vi "Current Elevator State.vi"(8 "error in (no error)":errorcluster, 10 "Elevator State":T1 {"Current Elevation" scale=0.0..100.0; "Current Travel Rate" scale=-1.0..1.0}, 11 "GTH-Assessing in":refnum<class "GTH-Assessing.lvclass">) -> (0 "error out":errorcluster, 3 "GTH-Assessing out":refnum<class "GTH-Assessing.lvclass">)   [LabVIEW 2014, in "Elevator.lvlib" / "EL-Go To Height.lvlib" / "GTH-Assessing.lvclass"]
uses:
  GTH-Assessing.lvclass
  Elevator Class/Elevator State.ctl
  <vilib>/ActorFramework/Actor/Actor.lvclass/Actor.ctl
  <vilib>/ActorFramework/Message Enqueuer/Message Enqueuer.lvclass/Message Enqueuer.ctl
  <vilib>/ActorFramework/Message Enqueuer/Init from Existing Queue.vi
  <vilib>/ActorFramework/Message Enqueuer/Enqueue.vi
  <vilib>/ActorFramework/Message Priority Queue/Priority Enqueue.vi
  <vilib>/ActorFramework/Message Enqueuer/Message Enqueuer.lvclass
  EL-Go To Height Messages/Go To Holding Msg/Go To Holding Msg.lvclass
  EL-Go To Height Messages/Go To Down Msg/Go To Down Msg.lvclass
  EL-Go To Height Messages/Go To Up Msg/Go To Up Msg.lvclass
  EL-Go To Height Class/EL-Go To Height.lvclass
  <vilib>/ActorFramework/Actor/Actor.lvclass
  Elevator Class/Elevator.lvclass
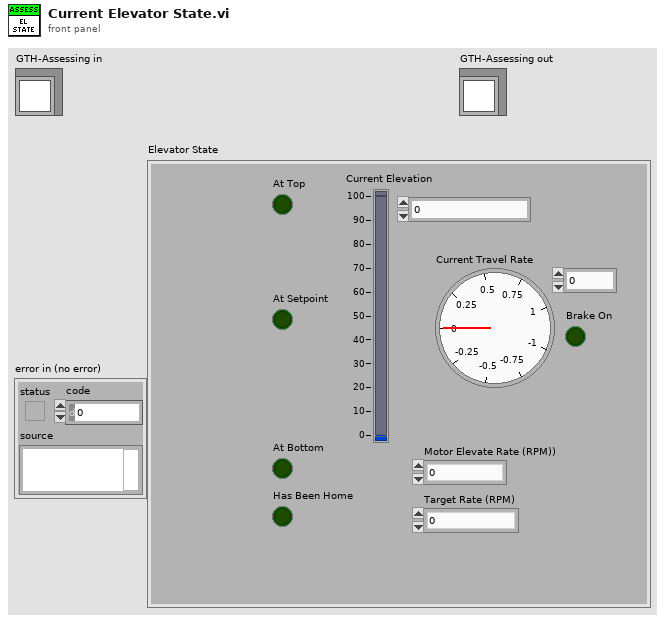
[diagram p1: front panel]
types:
  T1 = typedef "Elevator.lvlib/Elevator.lvclass/Elevator State.ctl" = cluster{"At Bottom":bool, "At Top":bool, "At Setpoint":bool, "Target Rate (RPM)":dbl, "Current Travel Rate":dbl, "Current Elevation":dbl, "Brake On":bool, "Motor Elevate Rate (RPM))":dbl, "Has Been Home":bool}
  T2 = typedef "Elevator.lvlib/EL-Go To Height.lvlib/EL-Go To Height.lvclass/Parameters.ctl" = cluster{"Target Height":dbl, "Elevator State Loop (ms)":u32, "Up Rate (Percentage)":dbl, "Down Rate (Percentage)":dbl}
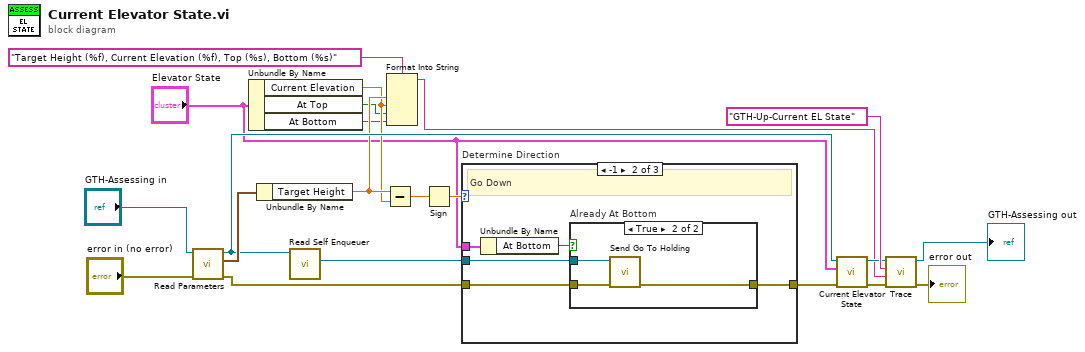
[diagram p0: block diagram]
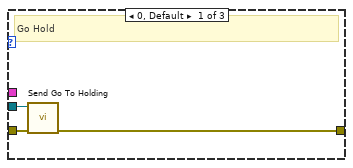
[diagram p2: hidden frame]
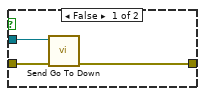
[diagram p3: hidden frame]
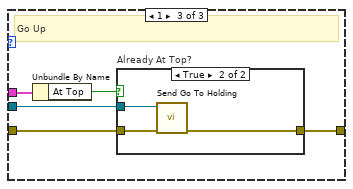
[diagram p4: hidden frame]
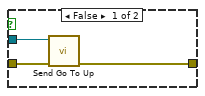
[diagram p5: hidden frame]
diagram:
  n1 = call-dynamic "Read Parameters.vi"("error in (no error)"="error in (no error)", "EL-Go To Height in"="GTH-Assessing in") -> ("error out"=w16:errorcluster, "Parameters"=w21:T2, "EL-Go To Height out"=w13:refnum<class "GTH-Assessing.lvclass">)  [unwired: 7 in]
  n2 = Unbundle By Name("Elevator State") -> ("Current Elevation"=w4:dbl, "At Top"=w2:bool, "At Bottom"=w1:bool)
  n3 = Unbundle By Name(w21) -> ("Target Height"=w5:dbl)
  n4 = call <vilib>:"Read Self Enqueuer.vi"("Actor"=w13) -> ("Self Enqueuer"=w18:refnum<class "Message Enqueuer.lvclass">)  [unwired: 10 in]
  n5 = Subtract(x=w5, y=w4) -> (x-y=w20:dbl)
  n6 = Format Into String(format string="Target Height (%f), Current Elevation (%f), Top (%s), Bottom (%s)", w5, w4, w2, w1) -> (resulting string=w6:string)  [unwired: 2 in, 1 out]
  n7 = Sign(1:w20) -> (0:w19:dbl)
  n8 = case "Determine Direction" shown="-1" w19 {
    tunnel: w18 -> [w24 w29 w38]
    tunnel: w16 -> [w23 w27 w37]
    tunnel: [w22 w28 w36] -> w15
    tunnel: "Elevator State" -> [_ w26 w40]
    frame 0, Default {
      # "Go Hold"
      n9 = call "Send Go To Holding.vi"("error in (no error)"=w23, "Message Enqueuer"=w24) -> ("error out"=w22:errorcluster)  [unwired: 8 in, 1 out]
    }
    frame -1 {
      # "Go Down"
      n10 = Unbundle By Name(w26) -> ("At Bottom"=w25:bool)
      n11 = case "Already At Bottom" shown="True" w25 {
        tunnel: w29 -> [w32 w34]
        tunnel: [w31 w33] -> w28
        tunnel: w27 -> [w30 w35]
        frame False {
          n12 = call "Send Go To Down.vi"("error in (no error)"=w30, "Message Enqueuer"=w32) -> ("error out"=w31:errorcluster)  [unwired: 8 in, 1 out]
        }
        frame True {
          n13 = call "Send Go To Holding.vi"("error in (no error)"=w35, "Message Enqueuer"=w34) -> ("error out"=w33:errorcluster)  [unwired: 8 in, 1 out]
        }
      }
    }
    frame 1 {
      # "Go Up"
      n14 = Unbundle By Name(w40) -> ("At Top"=w39:bool)
      n15 = case "Already At Top?" shown="True" w39 {
        tunnel: w38 -> [w43 w46]
        tunnel: w37 -> [w42 w45]
        tunnel: [w41 w44] -> w36
        frame False {
          n16 = call "Send Go To Up.vi"("error in (no error)"=w42, "Message Enqueuer"=w43) -> ("error out"=w41:errorcluster)  [unwired: 8 in, 1 out]
        }
        frame True {
          n17 = call "Send Go To Holding.vi"("error in (no error)"=w45, "Message Enqueuer"=w46) -> ("error out"=w44:errorcluster)  [unwired: 8 in, 1 out]
        }
      }
    }
  }
  n18 = call-parent "Current Elevator State.vi"("error in (no error)"=w15, "Elevator State"="Elevator State", "EL-Go To Height in"=w13) -> ("error out"=w11:errorcluster, "EL-Go To Height out"=w10:refnum<class "GTH-Assessing.lvclass">)  [unwired: 7 in]
  n19 = call-dynamic "Trace.vi"("error in (no error)"=w11, "Command Message"=w6, "Command Action"="GTH-Up-Current EL State", "Command Actor in"=w10) -> ("error out"=→"error out":errorcluster, "Command Actor out"=→"GTH-Assessing out":refnum<class "GTH-Assessing.lvclass">)  [unwired: 6 in]
